vi "Main.vi"() -> ()   [LabVIEW 2018, in "MQTT_Singleton.lvlib"]
doc: "This template is based off of the Queued Message Handler design pattern and the Queued Message Handler project template that ships with LabVIEW.\n\nThe main difference is that the queue is private to this module and communication between modules is performed via Broadcast and Request events.\n\nRequest events are wrapped in public API methods and are handled in the Event Handling Loop (EHL) of this VI. Any module can register for Broadcast events sent by this module. The EHL generates messages based on user interface actions.\n\nThe Message Handling Loop (MHL) processes messages generated by the EHL, or by other messages. The messages are string values, so new messages can be added easily to the Message Cases case structure in the MHL. Each message cluster can also provide an optional value for Message Data, which is a variant that can be converted to whatever message-specific data is required.\n_____\nBased on Delacor QMH Project Template 4.1.0.59."
uses:
  MQTT_Singleton.lvlib
  <vilib>/Delacor/Delacor QMH/Libraries/Module Admin_class/Delacor_lib_QMH_Module Admin.lvclass
  Module Data--cluster.ctl
  LVMQTT-master/Controls/Connection_Return_Codes.ctl
  AWS-IoT-RESTful-master/MQTT/Controls/ConnectMeta.ctl
  AWS-IoT-RESTful-master/MQTT/Controls/Retain_Flag.ctl
  AWS-IoT-RESTful-master/MQTT/Controls/DUP_Flag.ctl
  AWS-IoT-RESTful-master/MQTT/Controls/QoS.ctl
  AWS-IoT-RESTful-master/Controls/SSL_Connection.ctl
  Stop Argument--cluster.ctl
  <vilib>/Delacor/Delacor QMH/Libraries/Module Admin_class/Delacor_lib_QMH_Module Admin.lvclass/Delacor_lib_QMH_Module Admin.ctl
  Connect Argument--cluster.ctl
  Publish Argument--cluster.ctl
  Subscribe Argument--cluster.ctl
  Disconnect Argument--cluster.ctl
  <vilib>/Utility/miscctls.llb/LVPointTypeDef.ctl
  AWS-IoT-RESTful-master/MQTT/Controls/Connect_Flags.ctl
  AWS-IoT-RESTful-master/Controls/certs.ctl
  LVMQTT-master/Controls/QoS.ctl
  <vilib>/Delacor/Delacor QMH/Libraries/Module Admin_class/Delacor_lib_QMH_Get External Launch.vi
  HB.vi
  <vilib>/Delacor/Delacor QMH/Libraries/Message Queue_class/Delacor_lib_QMH_Enqueue Message (Single).vi
  <vilib>/Utility/error.llb/Error Cluster From Error Code.vi
  <vilib>/ErrorRing/Error Ring.xnode
  <vilib>/Delacor/Delacor QMH/Libraries/Message Queue_class/Delacor_lib_QMH_Message Queue.lvclass
  LVMQTT-master/MQTT_Functions.lvlib
  MQTT Messages.lvlib
  AWS-IoT-RESTful-master/AWS_IoT.lvlib
panel:
  out "Publish Message":string
  out "Publish Topic":string
  out "HB RX Count":u32
  out "Subscribe Topic":string
  out "Rx Message":string
  out "Rx Topic Name":string
  out "Latency (ms)":u32
  out "ms":u32
  out "HB TX Count":u32
  out "Acknowledged":bool
  out "error out":errorcluster
  in  "Module Admin":refnum<class "Delacor_lib_QMH_Module Admin.lvclass">
  out "Status":string
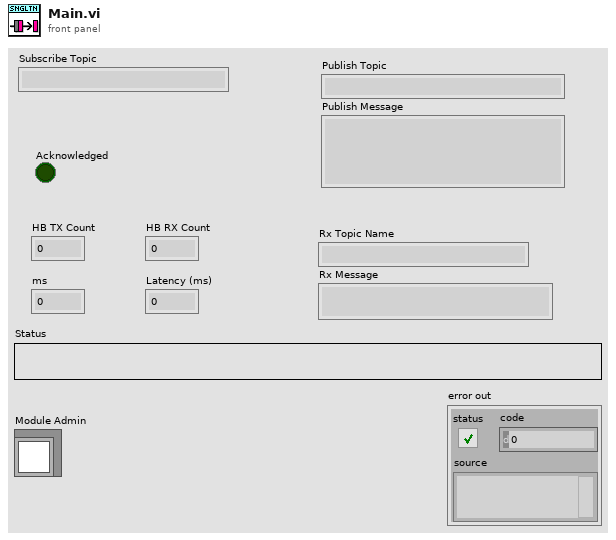
[diagram p1: front panel]
types:
  T1 = typedef "MQTT_Singleton.lvlib/Request Events--cluster.ctl" = cluster{"Stop Module":refnum<user-event>, "Show Panel":refnum<user-event>, "Hide Panel":refnum<user-event>, "Get Module Execution Status":refnum<user-event>, "Show Diagram":refnum<user-event>, "Connect":refnum<user-event>, "Publish":refnum<user-event>, "Subscribe":refnum<user-event>, "Disconnect":refnum<user-event>, "Start Listening":refnum<user-event>, "Stop Listening":refnum<user-event>, "Exit Listening":refnum<user-event>}
  T2 = typedef "MQTT_Singleton.lvlib/Module Data--cluster.ctl" = cluster{"Status":string, "Connection Status":T3, "Message ID":u16, "Listening?":bool, "Default Topics":string[], "Broker IP":string, "Client ID":string, "Connect Meta":T4, "SSL_Connection":T8, "CertPath":path, "KeyPath":path}
  T3 = typedef "MQTT_Functions.lvlib/Connection_Return_Codes.ctl" = enum16{"Connection accepted", "Connection refused: unacceptable protocol version", "Connection refused: identifier rejected", "Connection refused: Server unavailable", "Connection refused: bad user name or password", "Connection refused: not authorized"}
  T4 = typedef "AWS_IoT.lvlib/ConnectMeta.ctl" = cluster{"Retain":T5, "DUP":T6, "Keep Alive (sec)":u16, "QoS":T7}
  T5 = typedef "AWS_IoT.lvlib/Retain_Flag.ctl" = bool
  T6 = typedef "AWS_IoT.lvlib/DUP_Flag.ctl" = bool
  T7 = typedef "AWS_IoT.lvlib/QoS.ctl" = enum8{"At most once", "At least once", "Exactly once", "Reserved"}
  T8 = typedef "AWS_IoT.lvlib/SSL_Connection.ctl" = cluster{"connection ID":refnum<k5>, "TLS":cluster{"CXT ptr":i32, "SSL ptr":i32, "Socket ptr":i32}, "NIssleay library path":path, "server url":string}
  T9 = enum32{"invalid lock state", "Not Locked", "Locked (No Password)", "Password-protected"}
  T10 = typedef "MQTT_Singleton.lvlib/Stop Argument--cluster.ctl" = cluster{"Origin":string, "Exit via Stop Module Req?":bool, "Wait for Module to stop?":bool}
  T11 = typedef "MQTT_Singleton.lvlib/Connect Argument--cluster.ctl" = cluster{"Endpoint":string, "ClientID":string, "CertPath":path, "KeyPath":path}
  T12 = typedef "MQTT_Singleton.lvlib/Publish Argument--cluster.ctl" = cluster{"Topic":string, "Message":string}
  T13 = typedef "MQTT_Singleton.lvlib/Subscribe Argument--cluster.ctl" = cluster{"Topic":string}
  T14 = typedef "MQTT_Singleton.lvlib/Disconnect Argument--cluster.ctl" = cluster{"Disconnect?":bool}
  T15 = typedef "LVPointTypeDef.ctl" = cluster{"Horizontal":i16, "Vertical":i16}
  T16 = enum32{"Invalid", "Standard", "Closed", "Hidden", "Minimized", "Maximized"}
  T17 = typedef "AWS_IoT.lvlib/certs.ctl" = cluster{"client cert file":path, "client key file":path}
  T18 = typedef "AWS_IoT.lvlib/Connect_Flags.ctl" = cluster{"user name":bool, "password":bool, "will retain":bool, "will flag":bool, "clean session":bool, "reserved":bool, "will QoS":T7}
  T19 = typedef "MQTT_Functions.lvlib/QoS.ctl" = enum8{"At most once", "At least once", "Exactly once", "Reserved"}
  T20 = typedef "AWS_IoT.lvlib/Connection_Return_Codes.ctl" = enum16{"Connection accepted", "Connection refused: unacceptable protocol version", "Connection refused: identifier rejected", "Connection refused: Server unavailable", "Connection refused: bad user name or password", "Connection refused: not authorized"}
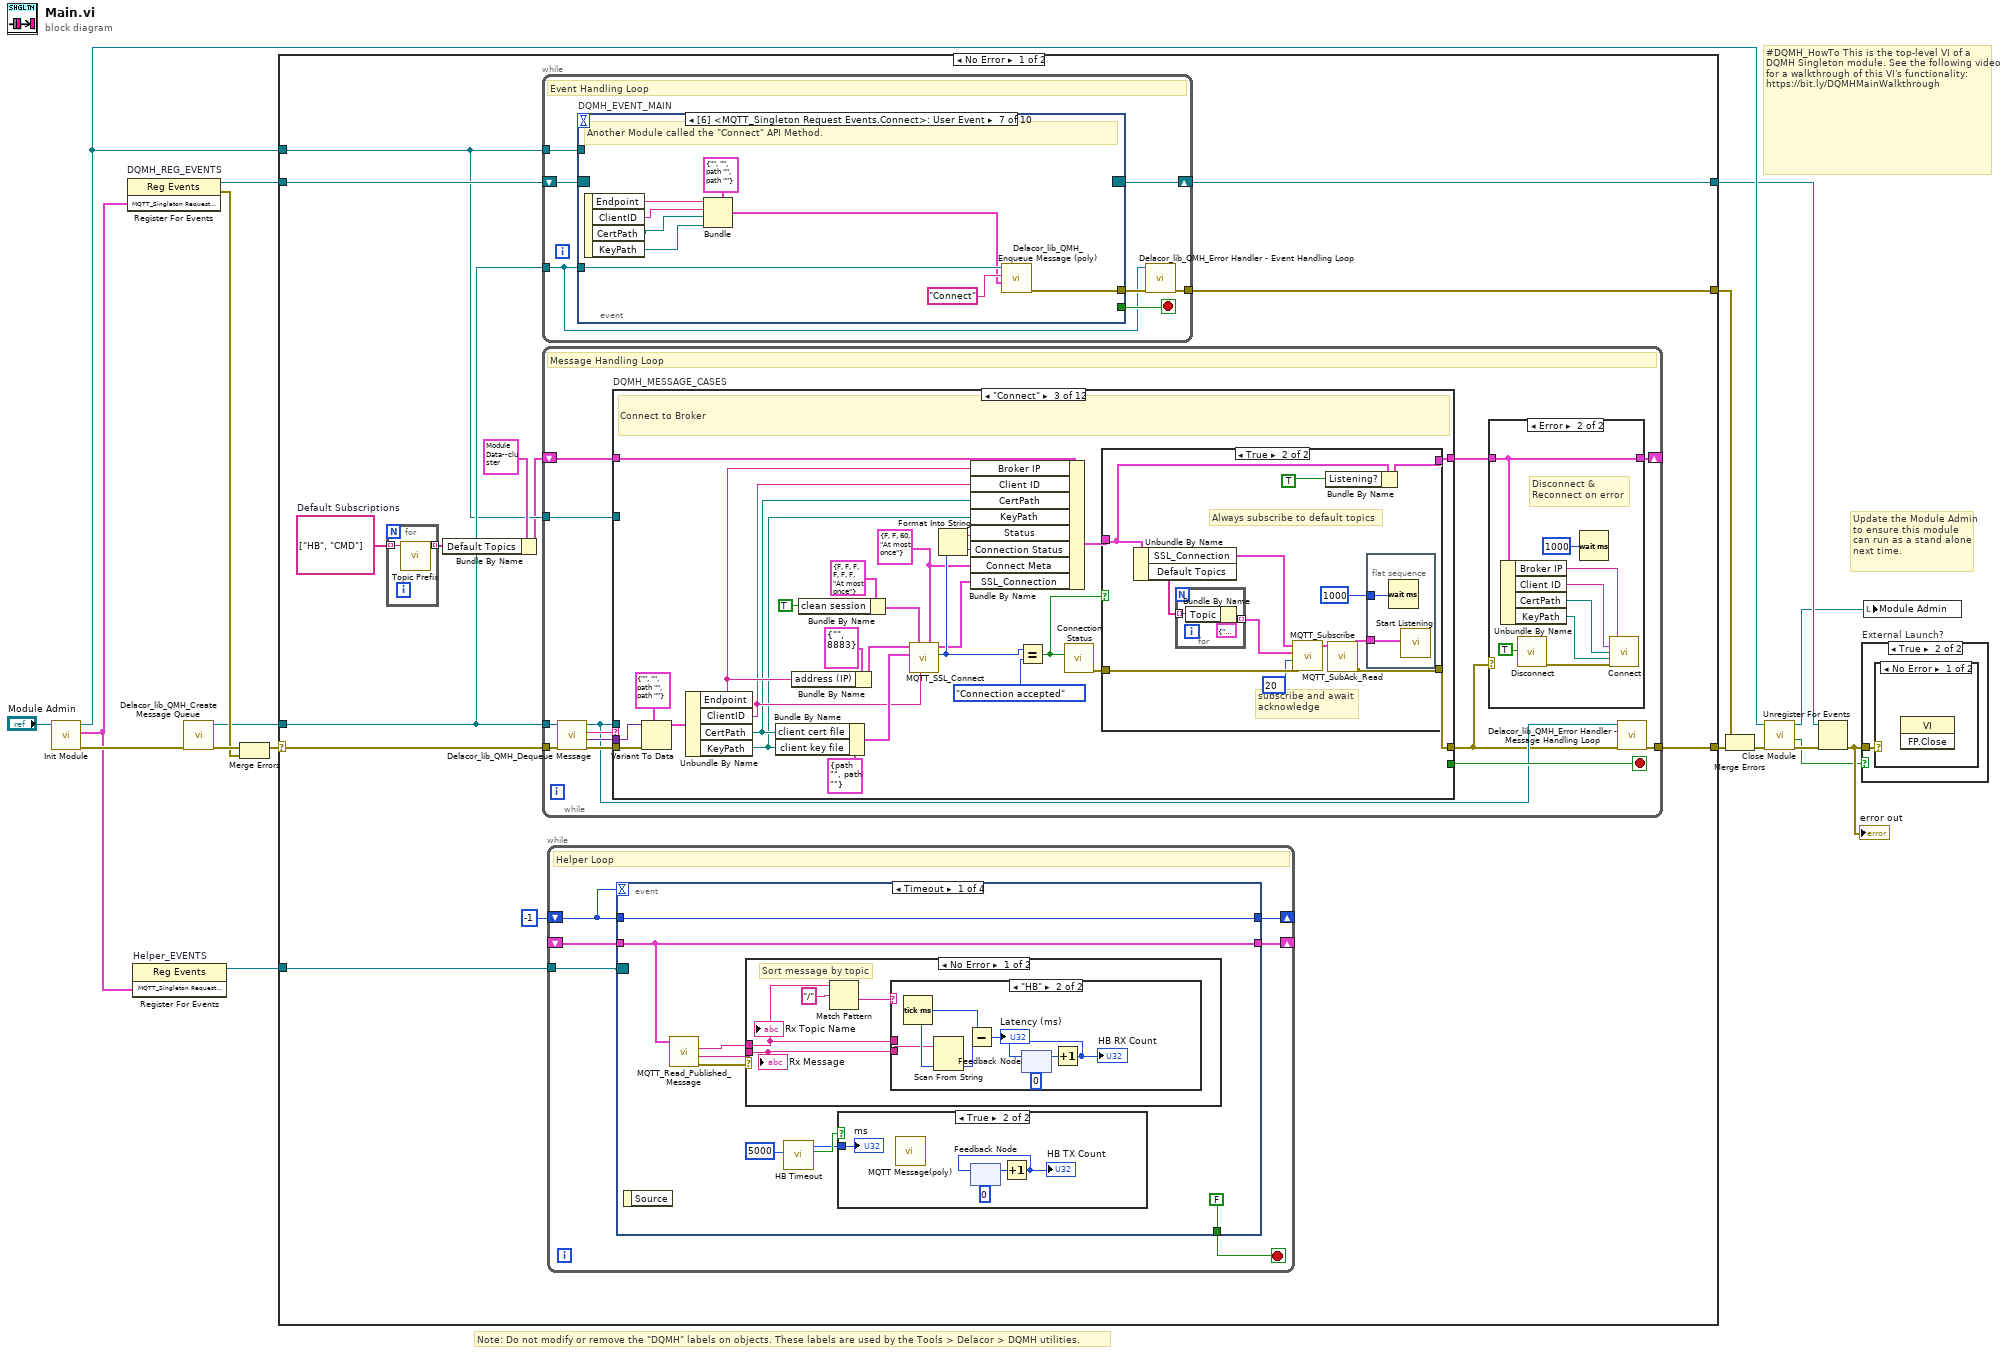
[diagram p0: block diagram]
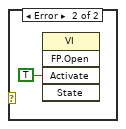
[diagram p3: hidden frame]
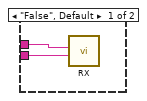
[diagram p5: hidden frame]
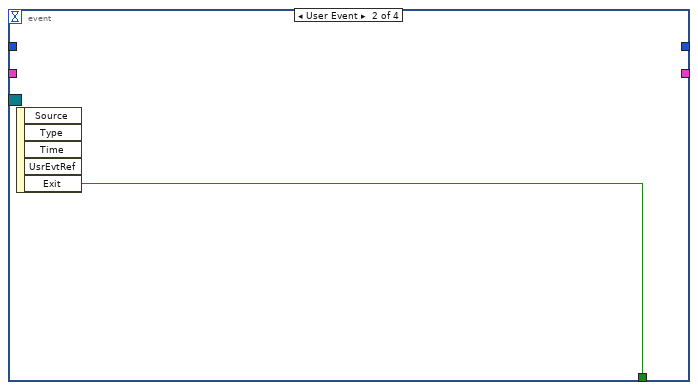
[diagram p7: hidden frame]
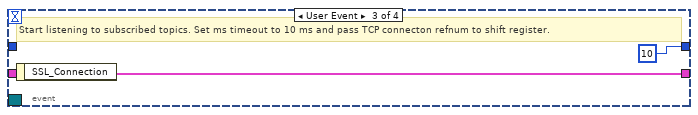
[diagram p8: hidden frame]
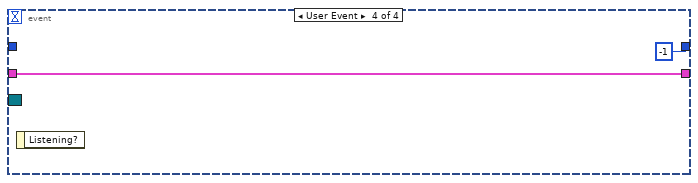
[diagram p9: hidden frame]
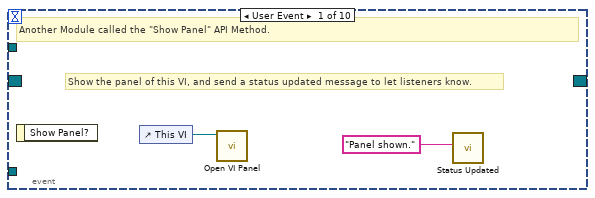
[diagram p10: hidden frame]
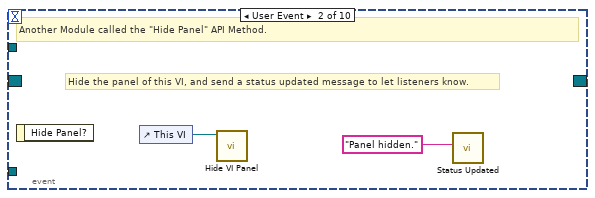
[diagram p11: hidden frame]
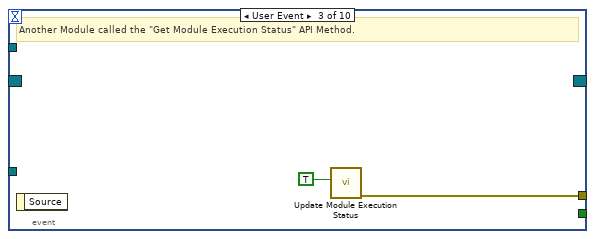
[diagram p12: hidden frame]
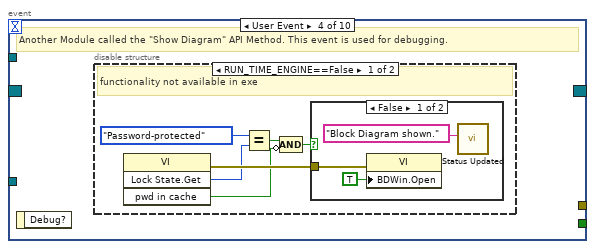
[diagram p13: hidden frame]
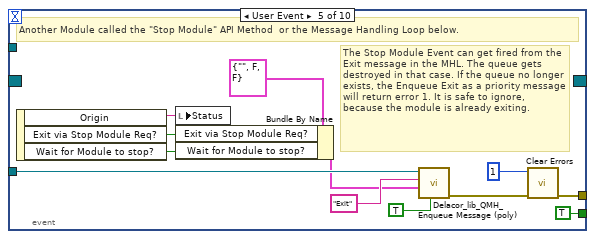
[diagram p16: hidden frame]
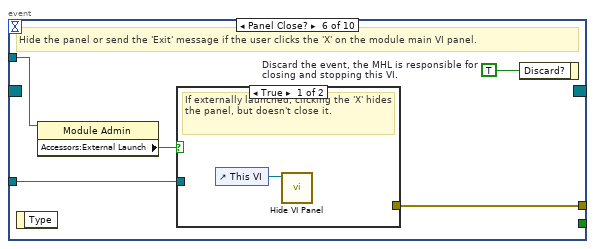
[diagram p17: hidden frame]
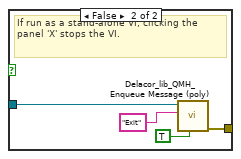
[diagram p18: hidden frame]
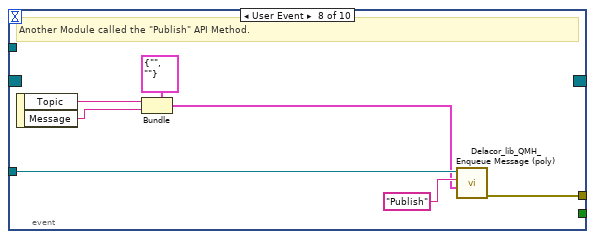
[diagram p19: hidden frame]
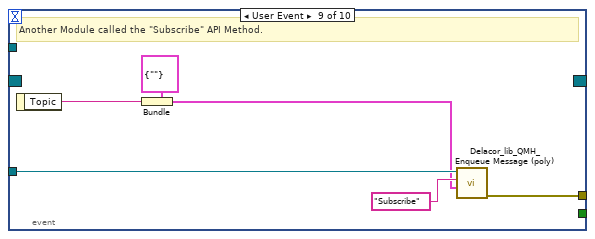
[diagram p20: hidden frame]
diagram:
  # "#DQMH_HowTo This is the top-level VI of a DQMH Singleton module. See the following video for a walkthrough of this VI's functionality: https://bit.ly/DQMHMainWalkthrough"
  # "Note: Do not modify or remove the \"DQMH\" labels on objects. These labels are used by the Tools > Delacor > DQMH utilities."
  # "Update the Module Admin to ensure this module can run as a stand alone next time."
  n1 = call "Init Module.vi"("Singleton Module Admin in"="Module Admin") -> ("error out"=w17:errorcluster, "MQTT_Singleton Request Events"=w2:T1, "Singleton Module Admin out"=w9:refnum<class "Delacor_lib_QMH_Module Admin.lvclass">)  [unwired: 8 in]
  n2 = register-events "DQMH_REG_EVENTS"(w2) -> (reference out=w7:refnum<event-registration>, error out=w10:errorcluster)  [unwired: 2 in]
  n3 = register-events "Helper_EVENTS"(w2) -> (reference out=w1:refnum<event-registration>)  [unwired: 2 in, 1 out]
  n4 = call <vilib>:"Delacor_lib_QMH_Create Message Queue.vi"("error in (no error)"=w17) -> ("error out"=w12:errorcluster, "Message Queue"=w6:refnum<class "Delacor_lib_QMH_Message Queue.lvclass">)  [unwired: 9 in]
  n5 = Merge Errors(w12, w10) -> (w11:errorcluster)
  n6 = case shown="No Error" w11 {
    selector: w11 -> [w29 w379]
    tunnel: [w31 w379] -> w18
    tunnel: [w28 w376] -> w8
    tunnel: w7 -> [w26 w376]
    tunnel: w6 -> [w25 _]
    tunnel: [w30 _] -> w15
    tunnel: w9 -> [w24 w372]
    tunnel: w1 -> [w22 _]
    frame No Error {
      w20 = string[] ["HB", "CMD"]  # Default Subscriptions
      n7 = for {
        tunnel: w20 -> [w33] mode=indexing
        tunnel: [w32] -> w19 mode=indexing
        n8 = call "Topic Prefix.vi"("Topic"=w33) -> ("Topic"=w32:string)  [unwired: 9 in, 1 out]
      }
      n9 = Bundle By Name(cluster=T2 {"Status"="", "Connection Status"=enum."Connection refused: not authorized", "Message ID"=10, "Listening?"=FALSE, "Default Topics"=[], "Broker IP"="", "Client ID"="", "Connect Meta"={"Retain"=FALSE, "DUP"=FALSE, "Keep Alive (sec)"=60, "QoS"=enum."At most once"}, "SSL_Connection"={"connection ID"=refnum, "TLS"={"CXT ptr"=0, "SSL ptr"=0, "Socket ptr"=0}, "NIssleay library path"=path "", "server url"=""}, "CertPath"=path "", "KeyPath"=path ""} ("Data Cluster"), "Default Topics"=w19) -> (w21:T2)
      n10 = while {
        tunnel: w25 -> [w71]
        shift-right: [w74] -> w28
        shift-left: w26 -> [w75]
        tunnel: [w76] -> w30
        tunnel: w24 -> [w72]
        stop <- w73 stop-if-true
        # "Event Handling Loop"
        n11 = event "DQMH_EVENT_MAIN" shown="[6] <MQTT_Singleton Request Events.Connect>: User Event" {
          selector: w75 -> [_ _ _ _ _ _ _ _ _ _]
          dyn-events: [_ _ _ _ _ _ _ _ _ _] -> w74
          timeout: _ -> [_ _ _ _ _ _ _ _ _ _]
          tunnel: [_ _ _ _ TRUE ("Discard?") _ _ _ _ _] -> w73
          tunnel: w71 -> [_ _ _ _ w100 w107 w123 w130 w136 w142]
          tunnel: [_ _ w83 _ w103 w109 w117 w124 w131 w137] -> w77
          tunnel: w72 -> [_ _ _ _ _ w106 _ _ _ _]
          event User Event {
            # "Show the panel of this VI, and send a status updated message to let listeners know."
            # "Another Module called the \"Show Panel\" API Method."
            n12 = event-data() -> ()  [unwired: 1 in, 1 out]
            n13 = control-ref of="This VI"() -> (w79:refnum<vi>)
            n14 = call "Open VI Panel.vi"("VI"=w79) -> ()  [unwired: 10 in, 1 out]
            n15 = call "Status Updated.vi"("Status"="Panel shown." ("format string")) -> ()  [unwired: 10 in, 1 out]
          }
          event User Event {
            # "Hide the panel of this VI, and send a status updated message to let listeners know."
            # "Another Module called the \"Hide Panel\" API Method."
            n16 = event-data() -> ()  [unwired: 1 in, 1 out]
            n17 = control-ref of="This VI"() -> (w81:refnum<vi>)
            n18 = call "Hide VI Panel.vi"("VI"=w81) -> ()  [unwired: 10 in, 1 out]
            n19 = call "Status Updated.vi"("Status"="Panel hidden." ("format string")) -> ()  [unwired: 10 in, 1 out]
          }
          event User Event {
            # "Another Module called the \"Get Module Execution Status\" API Method."
            n20 = event-data() -> ()  [unwired: 1 in, 1 out]
            n21 = call "Update Module Execution Status.vi"("Running?"=TRUE) -> ("error out"=w83:errorcluster)  [unwired: 10 in]
          }
          event User Event {
            # "Another Module called the \"Show Diagram\" API Method. This event is used for debugging."
            n22 = event-data() -> ()  [unwired: 1 in, 1 out]
            n23 = disable-structure shown="RUN_TIME_ENGINE==False" {
              frame condition #0 (active) {
                # "functionality not available in exe"
                n24 = invoke class="VI" method="Lock State.Get"() -> (error out=w89:errorcluster, "Get Lock State"=w88:T9, "pwd in cache"=w85:bool)  [unwired: 4 in, 1 out]
                n25 = Equal?(x=T9."Password-protected", y=w88) -> (x = y?=w86:bool)
                n26 = Compound Arithmetic op=AND(w86, invert w85) -> (w84:bool)
                n27 = case shown="False" w84 {
                  tunnel: w89 -> [w92 _]
                  frame False {
                    n28 = property class="VI"(error in=w92, "BDWin.Open"=TRUE ("Block Diagram Window:Open")) -> ()  [unwired: 1 in, 2 out]
                    n29 = call "Status Updated.vi"("Status"="Block Diagram shown." ("format string")) -> ()  [unwired: 10 in, 1 out]
                  }
                  frame True {
                    # "Password-protected VI, and the password is not in the cache. Do not show the diagram."
                  }
                }
              }
              frame condition #1 {
              }
            }
          }
          event User Event {
            # "The Stop Module Event can get fired from the Exit message in the MHL. The queue gets destroyed in that case. If the queue no longer exists, the Enqueue Exit as a priority message will return error 1. It is safe to ignore, because the module is already exiting."
            # "Another Module called the \"Stop Module\" API Method  or the Message Handling Loop below."
            n30 = event-data() -> ("Origin"=w99:string, "Exit via Stop Module Req?"=w95:bool, "Wait for Module to stop?"=w94:bool)  [unwired: 1 in]
            n31 = local write "Status"(w99) -> ()
            n32 = Bundle By Name(cluster=T10 {"Origin"="", "Exit via Stop Module Req?"=FALSE, "Wait for Module to stop?"=FALSE} ("Stop Argument"), "Exit via Stop Module Req?"=w95, "Wait for Module to stop?"=w94) -> (w93:T10)
            n33 = call-poly <vilib>:"Delacor_lib_QMH_Enqueue Message (poly).vi"("Priority Message? (F)"=TRUE, "Message Data"=w93, "Message"="Exit", "Message Queue in"=w100) -> ("error out"=w104:errorcluster)  [unwired: 6 in, 1 out]
            n34 = call <vilib>:"Clear Errors.vi"("error in (no error)"=w104, "specific error code to clear (0: all)"=1) -> ("error out"=w103:errorcluster)  [unwired: 4 in, 1 out]
          }
          event Panel Close? {
            w108 = TRUE  # Discard the event, the MHL is responsible for closing and stopping this VI.
            # "Hide the panel or send the 'Exit' message if the user clicks the 'X' on the module main VI panel."
            n35 = event-data() -> ()  [unwired: 1 in, 1 out]
            n36 = property class="Module Admin"(reference=w106) -> ("Accessors:External Launch"=w105:bool)  [unwired: 1 in, 2 out]
            n37 = case shown="True" w105 {
              tunnel: w107 -> [_ w113]
              tunnel: [_ w114] -> w109
              frame True {
                # "If externally launched, clicking the 'X' hides the panel, but doesn't close it."
                n38 = control-ref of="This VI"() -> (w110:refnum<vi>)
                n39 = call "Hide VI Panel.vi"("VI"=w110) -> ()  [unwired: 10 in, 1 out]
              }
              frame False {
                # "If run as a stand-alone VI, clicking the panel 'X' stops the VI."
                n40 = call-poly <vilib>:"Delacor_lib_QMH_Enqueue Message (poly).vi"("Priority Message? (F)"=TRUE, "Message"="Exit", "Message Queue in"=w113) -> ("error out"=w114:errorcluster)  [unwired: 7 in, 1 out]
              }
            }
            n41 = event-data("Discard?"=w108) -> ()  [unwired: 1 in, 1 out]
          }
          event User Event {
            # "Another Module called the \"Connect\" API Method."
            n42 = event-data() -> ("Endpoint"=w119:string, "ClientID"=w118:string, "CertPath"=w116:path, "KeyPath"=w115:path)  [unwired: 1 in]
            n43 = Bundle(cluster=T11 {"Endpoint"="", "ClientID"="", "CertPath"=path "", "KeyPath"=path ""} ("Connect Argument"), "Endpoint"=w119, "ClientID"=w118, "CertPath"=w116, "KeyPath"=w115) -> (w120:T11)
            n44 = call-poly <vilib>:"Delacor_lib_QMH_Enqueue Message (poly).vi"("Message Data"=w120, "Message"="Connect", "Message Queue in"=w123) -> ("error out"=w117:errorcluster)  [unwired: 7 in, 1 out]
          }
          event User Event {
            # "Another Module called the \"Publish\" API Method."
            n45 = event-data() -> ("Topic"=w126:string, "Message"=w125:string)  [unwired: 1 in]
            n46 = Bundle(cluster=T12 {"Topic"="", "Message"=""} ("Publish Argument"), "Topic"=w126, "Message"=w125) -> (w127:T12)
            n47 = call-poly <vilib>:"Delacor_lib_QMH_Enqueue Message (poly).vi"("Message Data"=w127, "Message"="Publish", "Message Queue in"=w130) -> ("error out"=w124:errorcluster)  [unwired: 7 in, 1 out]
          }
          event User Event {
            # "Another Module called the \"Subscribe\" API Method."
            n48 = event-data() -> ("Topic"=w132:string)  [unwired: 1 in]
            n49 = Bundle(cluster=T13 {"Topic"=""} ("Subscribe Argument"), "Topic"=w132) -> (w133:T13)
            n50 = call-poly <vilib>:"Delacor_lib_QMH_Enqueue Message (poly).vi"("Message Data"=w133, "Message"="Subscribe", "Message Queue in"=w136) -> ("error out"=w131:errorcluster)  [unwired: 7 in, 1 out]
          }
          event User Event {
            # "Another Module called the \"Disconnect\" API Method."
            n51 = event-data() -> ("Disconnect?"=w138:bool)  [unwired: 1 in]
            n52 = Bundle(cluster=T14 {"Disconnect?"=FALSE} ("Disconnect Argument"), "Disconnect?"=w138) -> (w139:T14)
            n53 = call-poly <vilib>:"Delacor_lib_QMH_Enqueue Message (poly).vi"("Message Data"=w139, "Message"="Disconnect", "Message Queue in"=w142) -> ("error out"=w137:errorcluster)  [unwired: 7 in, 1 out]
          }
        }
        n54 = call-dynamic "Delacor_lib_QMH_Error Handler - Event Handling Loop.vi"("error in (no error)"=w77, "Message Queue in"=w71) -> ("dup error in"=w76:errorcluster)  [unwired: 8 in, 1 out]
      }
      n55 = while {
        tunnel: w25 -> [w148]
        shift-right: [w144] -> _
        shift-left: w21 -> [w152]
        tunnel: w29 -> [w155]
        tunnel: [w153] -> w31
        tunnel: w24 -> [w146]
        stop <- w151 stop-if-true
        # "Message Handling Loop"
        n56 = call-dynamic "Delacor_lib_QMH_Dequeue Message.vi"("error in (no error)"=w155, "Message Queue in"=w148) -> ("error out"=w154:errorcluster, "Message Data"=w149:variant, "Message"=w150:string, "Message Queue out"=w147:refnum<class "Delacor_lib_QMH_Message Queue.lvclass">)  [unwired: 6 in]
        n57 = case "DQMH_MESSAGE_CASES" shown="\"Connect\"" w150 {
          selector: w150 -> [_ _ _ _ _ _ _ _ _ _ _ w359]
          tunnel: w147 -> [_ _ _ _ _ _ _ _ _ w327 w352 _]
          tunnel: w154 -> [w182 w186 w212 w250 w292 w306 w310 w312 w317 w334 w357 w361]
          tunnel: [w180 w186 w205 w235 w275 w299 w309 w312 w316 w330 w342 w362] -> w145
          tunnel: w152 -> [w171 w185 w211 w246 w288 w303 w308 w311 w314 w329 w351 w360]
          tunnel: [w170 w185 w201 w246 w284 w301 w308 w311 w314 w329 w351 w360] -> w143
          tunnel: [_ _ _ _ _ _ _ _ _ _ w344 _] -> w151
          tunnel: w149 -> [_ _ w210 w249 w291 w305 _ _ _ w328 w350 _]
          tunnel: w146 -> [w172 _ _ _ _ _ _ _ _ w326 w345 _]
          frame "Initialize" {
            w165 = "Initial Message" ("Initial Message")
            # "#CodeNeeded - Initialize the appearance of the front panel."
            # "#CodeNeeded - Initialize your state data here."
            # "Initialize - Any operation that needs to be done before the module can receive messages. Synchronize Caller Events.vi will inform Start Module.vi that the module has launched and is ready to receive messages. Module Did Init.vi will broadcast that the module initialized."
            n58 = call "Synchronize Caller Events.vi"("error in (no error)"=w182, "Singleton Module Admin in"=w172) -> ("error out"=w181:errorcluster, "Singleton Module Admin out"=w167:refnum<class "Delacor_lib_QMH_Module Admin.lvclass">)  [unwired: 8 in]
            n59 = property class="Module Admin"(reference=w167) -> ("Accessors:External Launch"=w176:bool)  [unwired: 1 in, 2 out]
            n60 = Select(t=T16."Hidden" ("State"), s=w176, f=T16."Standard" ("State")) -> (s? t:f=w173:T16)
            n61 = call "Module Name--constant.vi"() -> ("Module Name"=w179:string)  [unwired: 11 in]
            n62 = property class="VI"("Front Panel.Title"=w179) -> (reference out=w178:refnum<vi>, error out=w184:errorcluster)  [unwired: 2 in]
            n63 = call "Module Name--constant.vi"() -> ("Module Name"=w168:string)  [unwired: 11 in]
            n64 = invoke class="VI" method="FP.Open"(reference=w178, error in=w184, "State"=w173) -> (reference out=w177:refnum<vi>, error out=w183:errorcluster)  [unwired: 2 in, 3 out]
            n65 = Bundle By Name(cluster=w171, "Status"=w165) -> (w170:T2)
            n66 = call "Module Did Init.vi"("error in (no error)"=w181, "Initialized?"=TRUE, "Origin"=w168) -> ("error out"=w180:errorcluster)  [unwired: 8 in]
            n67 = invoke class="VI" method="FP.Center"(reference=w177, error in=w183) -> ()  [unwired: 1 in, 3 out]
            n68 = property on="Pane" class="Pane"("Origin"=T15 {"Horizontal"=0, "Vertical"=0}) -> ()  [unwired: 2 in, 2 out]
            "Status" <- w165
          }
          frame "--- Module Specific ---" {
            # "Separator -- The following cases handle messages specific to this Module."
          }
          frame "Connect" {
            w191 = T4 {"Retain"=FALSE, "DUP"=FALSE, "Keep Alive (sec)"=60, "QoS"=enum."At most once"} ("Connect Meta")
            # "Connect to Broker"
            n69 = Variant To Data(error in=w212, type=T11 {"Endpoint"="", "ClientID"="", "CertPath"=path "", "KeyPath"=path ""} ("Connect Argument"), Variant=w210) -> (data=w208:T11)  [unwired: 1 out]
            n70 = Unbundle By Name(w208) -> ("Endpoint"=w190:string, "ClientID"=w189:string, "CertPath"=w188:path, "KeyPath"=w187:path)
            n71 = Bundle By Name(cluster=T17 {"client cert file"=path "", "client key file"=path ""} ("cert path"), "client cert file"=w188, "client key file"=w187) -> (w194:T17)
            n72 = Bundle By Name(cluster=cluster{"address (IP)":string, "port":u16} {"address (IP)"="", "port"=8883} ("MQTT Broker"), "address (IP)"=w190) -> (w196:cluster{"address (IP)":string, "port":u16})
            n73 = Bundle By Name(cluster=T18 {"user name"=FALSE, "password"=FALSE, "will retain"=FALSE, "will flag"=FALSE, "clean session"=FALSE, "reserved"=FALSE, "will QoS"=enum."At most once"} ("Connect Flags"), "clean session"=TRUE) -> (w199:T18)
            n74 = call "MQTT_SSL_Connect.vi"("Connect Meta"=w191, "Client ID"=w189, "Connect Flags"=w199, "cert path"=w194, "MQTT Broker"=w196) -> ("Connection Status"=w193:T20, "SSL_Connection"=w192:T8)  [unwired: 4 in, 1 out]
            n75 = Format Into String(w193) -> (resulting string=w207:string)  [unwired: 3 in, 1 out]
            n76 = Bundle By Name(cluster=w211, "Broker IP"=w190, "Client ID"=w189, "CertPath"=w188, "KeyPath"=w187, "Status"=w207, "Connection Status"=w193, "Connect Meta"=w191, "SSL_Connection"=w192) -> (w202:T2)
            n77 = Equal?(x=w193, y=Connection_Return_Codes."Connection accepted" ("Connection Status")) -> (x = y?=w204:bool)
            n78 = call "Connection Status.vi"("Connection OK?"=w204) -> ("error out"=w203:errorcluster)  [unwired: 10 in]
            n79 = case shown="True" w204 {
              tunnel: [w214 w216] -> w205
              tunnel: w203 -> [w214 w220]
              tunnel: w202 -> [w213 w225]
              tunnel: [w213 w224] -> w201
              frame False {
              }
              frame True {
                # "Always subscribe to default topics"
                # "subscribe and await\nacknowledge"
                n80 = Unbundle By Name(w225) -> ("SSL_Connection"=w218:T8, "Default Topics"=w226:string[])
                n81 = for {
                  tunnel: w226 -> [w230] mode=indexing
                  tunnel: [w229] -> w219 mode=indexing
                  n82 = Bundle By Name(cluster=cluster{"Topic":string, "QoS":T19} {"Topic"="", "QoS"=enum."At most once"} ("Subscription Info"), "Topic"=w230) -> (w229:cluster{"Topic":string, "QoS":T19})
                }
                n83 = call "MQTT_Subscribe.vi"("error in (no error)"=w220, "Message ID"=u16 20, "Subscription Info Array"=w219, "SSL_Connection"=w218) -> ("SSL_Connection"=w221:T8)  [unwired: 6 in, 1 out]
                n84 = Bundle By Name(cluster=w225, "Listening?"=TRUE) -> (w224:T2)
                n85 = call "MQTT_SubAck_Read.vi"("SSL_Connection"=w221) -> ("error out"=w216:errorcluster, "SSL_Connection 2"=w215:T8)  [unwired: 8 in, 1 out]
                n86 = flat-sequence {
                  tunnel: w215 -> [w228]
                  tunnel: u32 1000 ("milliseconds to wait") -> [w227]
                  frame #0 {
                    n87 = Wait (ms)(milliseconds to wait=w227) -> ()  [unwired: 1 out]
                    n88 = call "Start Listening.vi"("SSL_Connection"=w228) -> ()  [unwired: 10 in, 1 out]
                  }
                }
              }
            }
          }
          frame "Publish" {
            # "Publish a message to the broker on a specific topic"
            n89 = Variant To Data(error in=w250, type=T12 {"Topic"="", "Message"=""} ("Publish Argument"), Variant=w249) -> (data=w247:T12, error out=w239:errorcluster)
            n90 = Unbundle By Name(w246) -> ("Connect Meta"=w245:T4, "SSL_Connection"=w243:T8)
            n91 = Unbundle By Name(w247) -> ("Topic"=w241:string, "Message"=w240:string)
            "Publish Topic" <- w241
            "Publish Message" <- w240
            n92 = Unbundle By Name(w245) -> ("QoS"=w242:T7)
            n93 = feedback #1(u16 10 ("Message ID")) -> (w244:u16)
            n94 = Increment(x=w244) -> (x+1=w238:u16)
            n95 = call "MQTT_SSL_Publish.vi"("Message ID"=w238, "error in (no error)"=w239, "Message to be published"=w240, "Topic"=w241, "SSL_Connection"=w243) -> ("error out"=w233:errorcluster, "SSL_Connection"=w232:T8)  [unwired: 5 in]
            n96 = case shown="\"At most once\", Default" w242 {
              tunnel: w233 -> [w253 w260 w272]
              tunnel: w232 -> [w254 w261 w273]
              tunnel: [w253 w258 w265] -> w235
              tunnel: [w254 w257 w266] -> _
              tunnel: w238 -> [w251 w259 w271]
              tunnel: [FALSE w256 w267] -> w236
              tunnel: [w251 w255 w264] -> w234
              frame "At most once", Default {
                # "QoS 0: no PubACK, fire and forget"
              }
              frame "At least once" {
                # "QoS 1: PubACK"
                n97 = call "MQTT_PubAck_Read.vi"("error in (no error)"=w260, "SSL_Connection"=w261) -> ("error out"=w258:errorcluster, "Message ID"=w255:u16, "SSL_Connection"=w257:T8)  [unwired: 7 in]
                n98 = Equal?(x=w255, y=w259) -> (x = y?=w256:bool)
              }
              frame "Exactly once" {
                # "QoS 2: PubREC, PubREL, PubCOMP"
                n99 = call "MQTT_PubRec_Read.vi"("error in (no error)"=w272, "SSL_Connection"=w273) -> ("error out"=w270:errorcluster, "Message ID"=w268:u16, "SSL_Connection"=w269:T8)  [unwired: 7 in]
                n100 = call "MQTT_PubRel_Send.vi"("error in (no error)"=w270, "Message ID"=w268, "SSL_Connection"=w269) -> ("error out"=w262:errorcluster, "SSL_Connection"=w263:T8)  [unwired: 6 in, 1 out]
                n101 = call "MQTT_PubComp_Read.vi"("error in (no error)"=w262, "SSL_Connection"=w263) -> ("error out"=w265:errorcluster, "Message ID"=w264:u16, "SSL_Connection"=w266:T8)  [unwired: 7 in]
                n102 = Equal?(x=w264, y=w271) -> (x = y?=w267:bool)
              }
            }
            "Acknowledged" <- w236
            n103 = feedback-in #1(w234) -> ()
          }
          frame "Subscribe" {
            # "Send the TCP connection info to the helper loop if listening? is F"
            # "subscribe and await\nacknowledge"
            # "Subscribe to a topic on the broker."
            n104 = Variant To Data(error in=w292, type=T13 {"Topic"=""} ("Subscribe Argument"), Variant=w291) -> (data=w289:T13, error out=w274:errorcluster)
            n105 = Unbundle By Name(w288) -> ("Listening?"=w285:bool, "SSL_Connection"=w277:T8, "Default Topics"=w282:string[])
            n106 = Unbundle By Name(w289) -> ("Topic"=w281:string)
            "Subscribe Topic" <- w281
            n107 = Build Array (concatenate)(w282, w281) -> (w280:string[])
            n108 = Bundle By Name(cluster=cluster{"Topic":string, "QoS":T19} {"Topic"="", "QoS"=enum."At most once"} ("Subscription Info"), "Topic"=w281) -> (w286:cluster{"Topic":string, "QoS":T19})
            n109 = Build Array(w286) -> (w278:cluster{"Topic":string, "QoS":T19}[])
            n110 = call "MQTT_Subscribe.vi"("error in (no error)"=w274, "Subscription Info Array"=w278, "SSL_Connection"=w277) -> ("SSL_Connection"=w279:T8)  [unwired: 7 in, 1 out]
            n111 = call "MQTT_SubAck_Read.vi"("SSL_Connection"=w279) -> ("error out"=w275:errorcluster, "SSL_Connection 2"=w276:T8)  [unwired: 8 in, 1 out]
            n112 = Bundle By Name(cluster=w288, "Listening?"=TRUE, "Default Topics"=w280) -> (w284:T2)
            n113 = case shown="False" w285 {
              tunnel: w276 -> [w294 _]
              frame False {
                n114 = call "Start Listening.vi"("SSL_Connection"=w294) -> ()  [unwired: 10 in, 1 out]
              }
              frame True {
              }
            }
            n115 = flat-sequence {
              tunnel: w275 -> [_]
              frame #0 {
                n116 = Wait (ms)(milliseconds to wait=u32 500) -> ()  [unwired: 1 out]
              }
            }
          }
          frame "Disconnect" {
            # "Disconnect from the broker."
            n117 = Variant To Data(error in=w306, type=T14 {"Disconnect?"=FALSE} ("Disconnect Argument"), Variant=w305) -> (error out=w296:errorcluster)  [unwired: 1 out]
            n118 = Unbundle By Name(w303) -> ("Listening?"=w302:bool, "SSL_Connection"=w297:T8)
            n119 = call "MQTT_SSL_Disconnect.vi"("error in (no error)"=w296, "SSL_Connection"=w297) -> ("error out"=w295:errorcluster)  [unwired: 9 in]
            n120 = case shown="True" w302 {
              selector: w302 -> [_ w307]
              frame False {
              }
              frame True {
                n121 = call "Stop Listening.vi"("Listening?"=w307) -> ()  [unwired: 10 in, 1 out]
              }
            }
            n122 = Bundle By Name(cluster=w303, "Listening?"=FALSE) -> (w301:T2)
            n123 = call "Connection Status.vi"("error in (no error)"=w295, "Connection OK?"=FALSE) -> ("error out"=w299:errorcluster)  [unwired: 9 in]
          }
          frame "---Copy This Frame---" {
            # "Duplicate this frame when creating new messages.  Change this comment in the duplicated frame to describe this message."
            n124 = Merge Errors(w310) -> (w309:errorcluster)
          }
          frame "--- Exit and Error Handling---" {
            # "Separator - The following cases handle errors and exit messages."
          }
          frame "Simulate MHL Error" {
            # "#DQMH_HowTo The 'Simulate MHL Error' button  illustrates how the MHL handles errors. This event is instructional in nature and can be removed."
            # "Simulate an error occurring at the MHL"
            n125 = call "Module Name--constant.vi"() -> ("Module Name"=w313:string)  [unwired: 11 in]
            n126 = xnode "Error Ring"("parameter 0"=w313) -> ("error out"=w315:errorcluster)
            n127 = Merge Errors(w317, w315) -> (w316:errorcluster)
          }
          frame "Error" {
            # "#CodeRecommended - If you ever change the name of this \"Error\" message, you'll need to update the name in the Check Loop Error.vi as well."
            # "#CodeRecommended - If the module is running in standalone mode (External Launch = FALSE), this code will pop up an error dialog and call the 'Exit' message if an error occurs. Add more fine-grained error handling here."
            # "Error - Check the error message data and respond accordingly. This message is sent by the \"Error Handler\" VIs at the end of each loop in this application."
            n128 = property class="Module Admin"(reference=w326) -> ("Accessors:External Launch"=w325:bool)  [unwired: 1 in, 2 out]
            n129 = Variant To Data(error in=w334, type=errorcluster {"status"=FALSE, "code"=0, "source"=""} ("error constant"), Variant=w328) -> (data=w335:errorcluster, error out=w332:errorcluster)
            n130 = call "Error Reported.vi"("Error"=w335) -> ()  [unwired: 10 in, 1 out]
            n131 = case shown="False" w325 {
              tunnel: [w340 _] -> w331
              tunnel: w327 -> [w338 _]
              tunnel: w335 -> [w339 _]
              frame False {
                # "If the module is running standalone, then pop up an error dialog and call the \"Exit\" message."
                n132 = call <vilib>:"Simple Error Handler.vi"("error in (no error)"=w339) -> ()  [unwired: 4 in, 5 out]
                n133 = call-poly <vilib>:"Delacor_lib_QMH_Enqueue Message (poly).vi"("Priority Message? (F)"=TRUE, "Message"="Exit", "Message Queue in"=w338) -> ("error out"=w340:errorcluster)  [unwired: 7 in, 1 out]
              }
              frame True {
                # "If the module was launched externally, calling the Error Reported broadcast VI is the only action performed by the \"Error\" message. The module's caller can then process the error appropriately."
              }
            }
            n134 = Merge Errors(w332, w331) -> (w330:errorcluster)
            n135 = local write "error out"(w330) -> ()
          }
          frame "Exit" {
            w349 = 91  # 91: not all Exit messages will have an argument
            w344 = TRUE  # Stop the VI
            # "Release the message queue reference"
            # "#CodeNeeded - Add any required cleanup code here"
            # "Exit - Exit the application."
            n136 = Variant To Data(error in=w357, type=T10 {"Origin"="", "Exit via Stop Module Req?"=FALSE, "Wait for Module to stop?"=FALSE} ("Stop Argument"), Variant=w350) -> (data=w347:T10, error out=w354:errorcluster)
            n137 = call <vilib>:"Clear Errors.vi"("error in (no error)"=w354, "specific error code to clear (0: all)"=w349) -> ("error out"=w356:errorcluster)  [unwired: 4 in, 1 out]
            n138 = control-ref of="This VI"() -> (w346:refnum<vi>)
            n139 = call-dynamic "Delacor_lib_QMH_Release Message Queue.vi"("error in (no error)"=w356, "Message Queue"=w352) -> ("error out"=w355:errorcluster)  [unwired: 9 in]
            n140 = call "Handle Exit.vi"("Stop Argument"=w347, "Admin in"=w345, "VI reference"=w346) -> ("error out"=w353:errorcluster)  [unwired: 7 in, 1 out]
            n141 = Merge Errors(w355, w353) -> (w343:errorcluster)
            n142 = call "Connection Status.vi"("error in (no error)"=w343, "Connection OK?"=FALSE) -> ("error out"=w342:errorcluster)  [unwired: 9 in]
            n143 = call "Exit Listening.vi"("Exit"=w344) -> ()  [unwired: 10 in, 1 out]
          }
          frame Default {
            # "'Default' case only runs if there is a message that isn't defined in any of the other cases.  Output a programming error."
            n144 = call "Module Name--constant.vi"() -> ("Module Name"=w358:string)  [unwired: 11 in]
            n145 = xnode "Error Ring"("parameter 0"=w359, "parameter 1"=w358) -> ("error out"=w363:errorcluster)
            n146 = Merge Errors(w361, w363) -> (w362:errorcluster)
          }
        }
        n147 = case shown="Error" w145 {
          tunnel: [w156 w163] -> w144
          tunnel: w143 -> [w156 w163]
          frame No Error {
          }
          frame Error {
            # "Disconnect &\nReconnect on error"
            n148 = Unbundle By Name(w163) -> ("Broker IP"=w162:string, "Client ID"=w161:string, "CertPath"=w158:path, "KeyPath"=w157:path)
            n149 = call "Disconnect.vi"("Disconnect?"=TRUE) -> ("error out"=w164:errorcluster)  [unwired: 10 in]
            n150 = Wait (ms)(milliseconds to wait=u32 1000) -> ()  [unwired: 1 out]
            n151 = call "Connect.vi"("Broker IP"=w162, "ClientID"=w161, "CertPath"=w158, "KeyPath"=w157, "error in (no error)"=w164) -> ()  [unwired: 10 in, 1 out]
          }
        }
        n152 = call-dynamic "Delacor_lib_QMH_Error Handler - Message Handling Loop.vi"("error in (no error)"=w145, "Message Queue in"=w147) -> ("dup error in"=w153:errorcluster)  [unwired: 8 in, 1 out]
      }
      n153 = while {
        shift-right: [w39] -> _
        shift-left: -1 -> [w38]
        tunnel: w22 -> [w36]
        shift-right: [w35] -> _
        shift-left: _ -> [w34]
        stop <- w37 stop-if-true
        # "Helper Loop"
        n154 = event shown="[0] Timeout" {
          selector: w36 -> [_ _ _ _]
          dyn-events: _ -> [_ _ _ _]
          timeout: w38 -> [_ _ _ _]
          tunnel: [w48 _ 10 -1] -> w39
          tunnel: w38 -> [w48 _ _ _]
          tunnel: [FALSE w66 _ _] -> w37
          tunnel: [w43 _ w68 w69] -> w35
          tunnel: w34 -> [w43 _ _ w69]
          event Timeout {
            n155 = event-data() -> ()  [unwired: 1 in, 1 out]
            n156 = call "MQTT_Read_Published_Message.vi"("SSL_Connection"=w43) -> ("error out"=w41:errorcluster, "Message"=w40:string, "Topic Name"=w42:string)  [unwired: 5 in, 3 out]
            n157 = case shown="No Error" w41 {
              tunnel: w42 -> [w54 _]
              tunnel: w40 -> [w53 _]
              frame No Error {
                # "Sort message by topic"
                n158 = Match Pattern(string=w54, regular expression="/") -> (after substring=w55:string)  [unwired: 1 in, 3 out]
                n159 = case shown="\"HB\"" w55 {
                  tunnel: w54 -> [w58 _]
                  tunnel: w53 -> [w57 w62]
                  frame "False", Default {
                    n160 = call "RX.vi"("Message"=w57, "Topic"=w58) -> ()  [unwired: 9 in, 1 out]
                  }
                  frame "HB" {
                    n161 = Tick Count (ms)() -> (millisecond timer value=w64:u32)
                    n162 = Scan From String(input string=w62, default 1=w64) -> (output 1=w65:u32)  [unwired: 3 in, 3 out]
                    n163 = Subtract(x=w64, y=w65) -> (x-y=→"Latency (ms)":u32)
                    n164 = feedback #2(u32 0 ("s? t:f")) -> (w60:u32)
                    n165 = Increment(x=w60) -> (x+1=w59:u32)
                    "HB RX Count" <- w59
                    n166 = feedback-in #2(w59) -> ()
                  }
                }
                "Rx Topic Name" <- w54
                "Rx Message" <- w53
              }
              frame Error {
              }
            }
            n167 = call "HB Timeout.vi"("HB Timeout ms"=u32 5000) -> ("Timeout"=w46:bool, "millisecond timer value"=w45:u32)  [unwired: 9 in]
            n168 = case shown="True" w46 {
              tunnel: w45 -> [_ w49]
              frame False {
              }
              frame True {
                n169 = call-poly "MQTT Message(poly).vi"() -> ()  [unwired: 11 in, 1 out]
                n170 = feedback #3(u32 0 ("s? t:f")) -> (w51:u32)
                n171 = Increment(x=w51) -> (x+1=w50:u32)
                "HB TX Count" <- w50
                n172 = feedback-in #3(w50) -> ()
                "ms" <- w49
              }
            }
          }
          event User Event {
            n173 = event-data() -> ("Exit"=w66:bool)  [unwired: 1 in, 4 out]
          }
          event User Event {
            # "Start listening to subscribed topics. Set ms timeout to 10 ms and pass TCP connecton refnum to shift register."
            n174 = event-data() -> ("SSL_Connection"=w68:T8)  [unwired: 1 in]
          }
          event User Event {
            n175 = event-data() -> ()  [unwired: 1 in, 1 out]
          }
        }
      }
    }
    frame Error {
      # "Synchronize Caller Events.vi will inform Start Module.vi that the module has launched and will let the code calling Start Module.vi register for broadcasts and would permit the caller receive the broadcast that an error occurred at launch time."
      n176 = call "Synchronize Caller Events.vi"("Singleton Module Admin in"=w372) -> ("error out"=w377:errorcluster)  [unwired: 9 in, 1 out]
      n177 = call "Module Name--constant.vi"() -> ("Module Name"=w375:string)  [unwired: 11 in]
      n178 = Format Into String(format string="An error occurred during initialization. %s is no longer running.", w375) -> (resulting string=w373:string)  [unwired: 2 in, 1 out]
      n179 = Merge Errors(w379, w377) -> (w378:errorcluster)
      n180 = call "Error Reported.vi"("Additional Information"=w373, "Error"=w378) -> ()  [unwired: 9 in, 1 out]
    }
  }
  n181 = Merge Errors(w15, w18) -> (w14:errorcluster)
  n182 = call "Close Module.vi"("error in (no error)"=w14, "Module Admin in"=w9) -> ("error out"=w16:errorcluster, "External Launch"=w3:bool, "Module Admin out"=w4:refnum<class "Delacor_lib_QMH_Module Admin.lvclass">)  [unwired: 7 in]
  n183 = Unregister For Events(event registration refnum=w8, error in=w16) -> (error out=w13:errorcluster)
  "error out" <- w13
  n184 = case "External Launch?" shown="True" w3 {
    tunnel: w13 -> [_ w380]
    frame False {
    }
    frame True {
      n185 = case shown="No Error" w380 {
        frame No Error {
          n186 = invoke class="VI" method="FP.Close"() -> ()  [unwired: 3 in, 3 out]
        }
        frame Error {
          n187 = invoke class="VI" method="FP.Open"("Activate"=TRUE ("Activate?")) -> ()  [unwired: 4 in, 5 out]
        }
      }
    }
  }
  n188 = local write "Module Admin"(w4) -> ()
